vi "RegisterBroadcastCallback.vi"(8 "error in (no error)":errorcluster, 9 "instance subscriber":bool, 10 "broadcast message":string, 11 "service in":refnum<class "IcmMessageService.lvclass">) -> (0 "error out":errorcluster, 3 "service out":refnum<class "IcmMessageService.lvclass">)   [LabVIEW 2017, in "IcmMessageService.lvclass"]
doc: "Subscribes the service to receive a particular type of message from the message bus callback whenever another service broadcasts that message. Ensure this VI runs prior to registering a callback for the message bus with the Register Callback VI."
uses:
  <vilib>/addons/InsightCM/MessageBus/MessageService/IcmMessageService.lvclass
  <vilib>/addons/InsightCM/MessageBus/MessageService/IcmMessageService.lvclass/IcmMessageService.ctl
  C:/Program Files (x86)/National Instruments/LabVIEW 2017/vi.lib/addons/InsightCM/Binaries/LabviewMessageAdapter.dll
  Binaries/LabviewMessageAdapter.dll
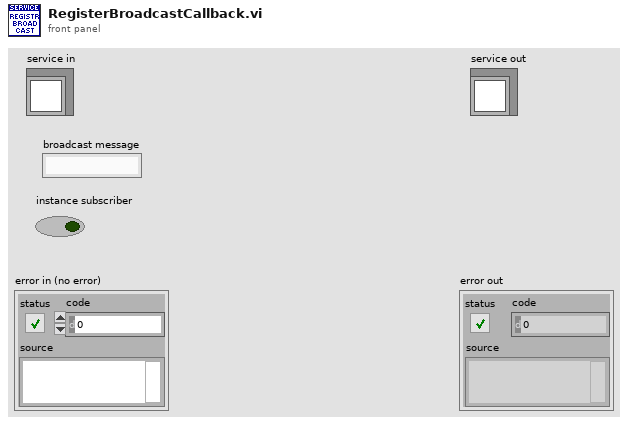
[diagram p1: front panel]
types:
  T1 = typedef "MessageServiceDvr.ctl" = refnum<data-value>
  T2 = typedef "MessageServiceData.ctl" = cluster{"Service":refnum<k24>}
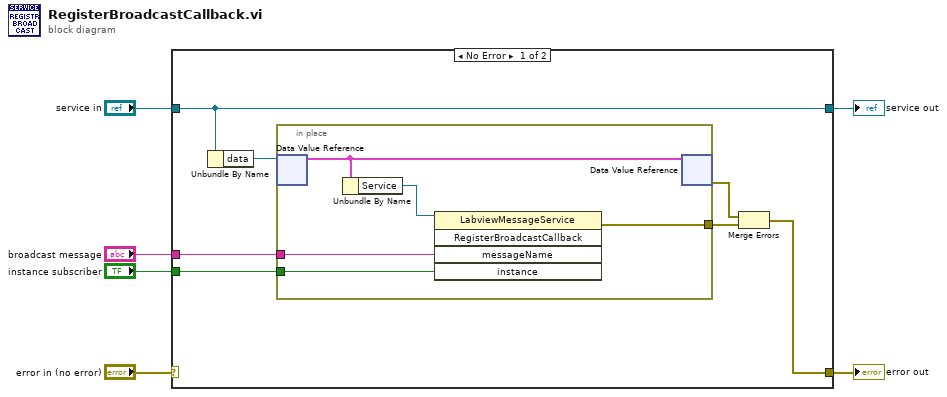
[diagram p0: block diagram]
diagram:
  n1 = case shown="No Error" "error in (no error)" {
    selector: "error in (no error)" -> [_ w20]
    tunnel: [w9 w20] -> w6
    tunnel: [w13 w19] -> w4
    tunnel: "service in" -> [w13 w19]
    tunnel: "broadcast message" -> [w8 _]
    tunnel: "instance subscriber" -> [w7 _]
    frame No Error {
      n2 = Unbundle By Name(w13) -> ("data"=w12:T1)
      n3 = in-place {
        in-place-border: [w17] -> w10
        in-place-border: w8 -> [w15]
        in-place-border: w7 -> [w14]
        n4 = in-place-dvr #1(w12) -> (w18:T2)  [unwired: 1 out]
        n5 = Unbundle By Name(w18) -> ("Service"=w16:refnum<k24>)
        n6 = invoke class="LabviewMessageService" method="RegisterBroadcastCallback"(reference=w16, "messageName"=w15, "instance"=w14) -> (error out=w17:errorcluster)  [unwired: 2 in, 4 out]
        n7 = in-place-dvr #1(w18) -> (w11:errorcluster)  [unwired: 1 out]
      }
      n8 = Merge Errors(w11, w10) -> (w9:errorcluster)
    }
    frame Error {
    }
  }
  "error out" <- w6
  "service out" <- w4
